vi "LoadDll.vi"(8 "error in (no error)":errorcluster) -> (0 "error out":errorcluster)   [LabVIEW 2020, in "FaceRecognitionDotNet.lvlib" / "FaceRecognition.lvclass"]
uses:
  FaceRecognition.lvclass
  dll/DlibDotNet.dll
  dll/FaceRecognitionDotNet.dll
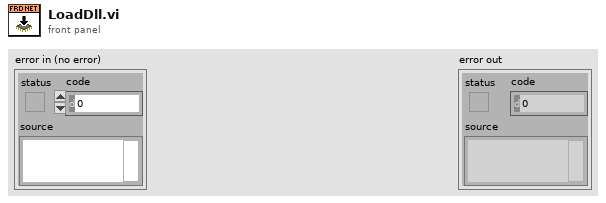
[diagram p1: front panel]
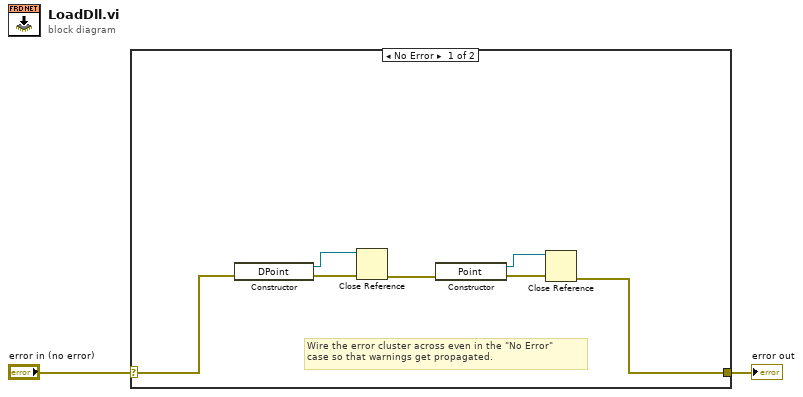
[diagram p0: block diagram]
diagram:
  n1 = case shown="No Error" "error in (no error)" {
    selector: "error in (no error)" -> [w4 w10]
    tunnel: [w3 w10] -> w1
    frame No Error {
      # "Wire the error cluster across even in the \"No Error\"\ncase so that warnings get propagated."
      n2 = constructor class="DPoint"(error in=w4) -> (reference out=w8:refnum<k24>, error out=w9:errorcluster)  [unwired: 2 in, 1 out]
      n3 = Close Reference(reference=w8, error in (no error)=w9) -> (error out=w5:errorcluster)
      n4 = constructor class="Point"(error in=w5) -> (reference out=w6:refnum<k24>, error out=w7:errorcluster)  [unwired: 2 in, 1 out]
      n5 = Close Reference(reference=w6, error in (no error)=w7) -> (error out=w3:errorcluster)
    }
    frame Error {
    }
  }
  "error out" <- w1
